vi "Draw_Cage_Outline_(sociability maze).vi"(0 "Picture refnum in":T2, 1 "Bounding rectangle for cage outline, pix (minor)":T1, 2 "Background color":u32(colorbox)=13816530, 3 "Error In":errorcluster) -> (5 "Picture refnum out":T2, 7 "Error Out":errorcluster)   [LabVIEW 2018, in "Cage Diagram.lvlib"]
uses:
  Cage Diagram.lvlib
  <vilib>/vision/Image Controls.llb/IMAQ Image.ctl
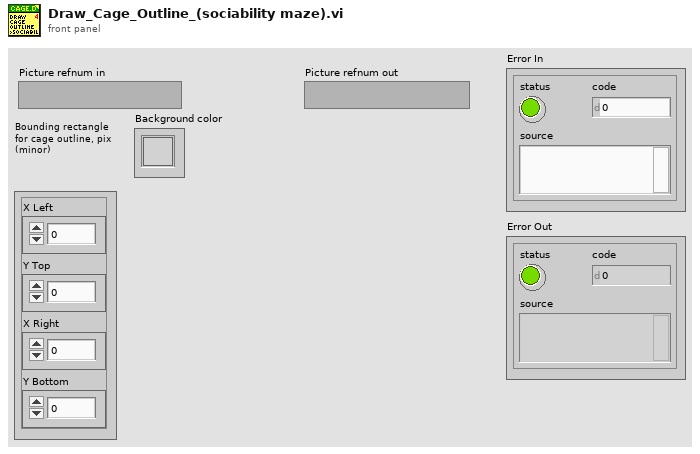
[diagram p1: front panel]
types:
  T1 = cluster{"X Left":i32, "Y Top":i32, "X Right":i32, "Y Bottom":i32}
  T2 = typedef "IMAQ Image.ctl" = refnum<image>
  T3 = cluster{"X Left":dbl, "Y Top":dbl, "X Right":dbl, "Y Bottom":dbl}
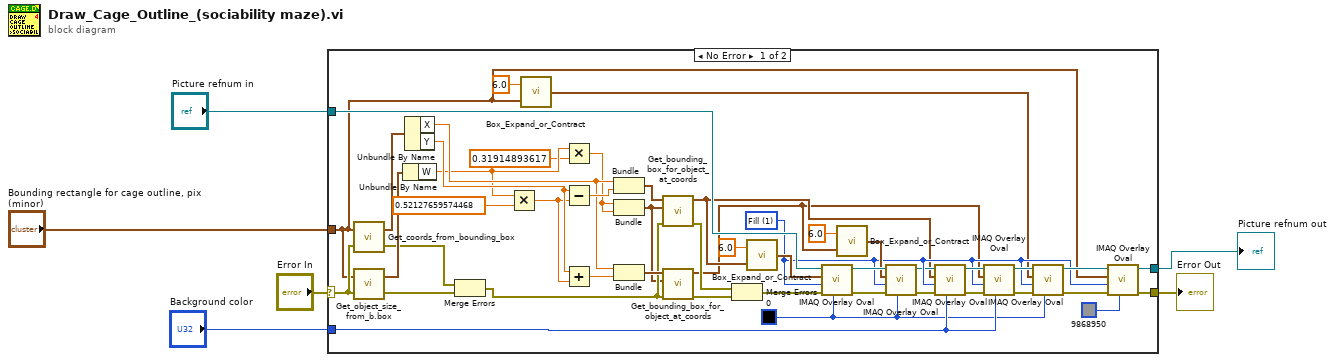
[diagram p0: block diagram]
diagram:
  n1 = case shown="No Error" "Error In" {
    selector: "Error In" -> [w44 w54]
    tunnel: [w28 w55] -> w5
    tunnel: "Picture refnum in" -> [w34 w55]
    tunnel: [w23 w54] -> w3
    tunnel: "Background color" -> [w12 _]
    tunnel: "Bounding rectangle for cage outline, pix (minor)" -> [w7 _]
    frame No Error {
      w9 = u32 0 ("Color")
      w14 = u32 1 items=["Frame", "Fill"] ("Drawing Mode (Frame)")
      n2 = call "Get_coords_from_bounding_box.vi"("Error In"=w44, "Object Bounding Box"=w7) -> ("Error Out"=w43:errorcluster, "Object Coords (center)"=w52:cluster{"X":dbl, "Y":dbl})
      n3 = call "Get_object_size_from_b.box.vi"("Error In"=w44, "Bounding rectangle for cage outline, pix"=w7) -> ("Error Out"=w42:errorcluster, "Object Size, pix"=w53:cluster{"W":dbl, "H":dbl})
      n4 = Unbundle By Name(w53) -> ("W"=w40:dbl)
      n5 = Unbundle By Name(w52) -> ("X"=w45:dbl, "Y"=w50:dbl)
      n6 = Merge Errors(w43, w42) -> (w41:errorcluster)
      n7 = Multiply(x=w40, y=0.52127659574468) -> (x*y=w18:dbl)
      n8 = call "Box_Expand_or_Contract.vi"("Rectangle in"=w7, "Expand/Contract"=6.0) -> ("Rectangle out"=w8:T3)
      n9 = Multiply(x=w40, y=0.31914893617) -> (x*y=w38:dbl)
      n10 = Subtract(x=w50, y=w18) -> (x-y=w49:dbl)
      n11 = Add(x=w50, y=w18) -> (x+y=w46:dbl)
      n12 = Bundle("X"=w45, w49) -> (w48:cluster{"X":dbl, dbl})  [unwired: 1 in]
      n13 = Bundle(w38, w38) -> (w37:cluster{dbl, dbl})  [unwired: 1 in]
      n14 = Bundle("X"=w45, w46) -> (w47:cluster{"X":dbl, dbl})  [unwired: 1 in]
      n15 = call "Get_bounding_box_for_object_at_coords.vi"("Error In"=w41, "Object Size, pix"=w37, "Object Coords, pix"=w48) -> ("Error Out"=w36:errorcluster, "Object Bounding Box"=w11:T3)  [unwired: 7 in]
      n16 = call "Get_bounding_box_for_object_at_coords.vi"("Error In"=w41, "Object Size, pix"=w37, "Object Coords, pix"=w47) -> ("Error Out"=w35:errorcluster, "Object Bounding Box"=w10:T3)  [unwired: 7 in]
      n17 = Merge Errors(w36, w35) -> (w33:errorcluster)
      n18 = call "Box_Expand_or_Contract.vi"("Rectangle in"=w11, "Expand/Contract"=6.0) -> ("Rectangle out"=w17:T3)
      n19 = call "IMAQ Overlay Oval"("Color"=w9, "error in (no error)"=w33, "Drawing Mode (Frame)"=w14, "Bounding Rectangle"=w17, "Image"=w34) -> ("error out"=w27:errorcluster, "Image Out"=w32:T2)  [unwired: 5 in]
      n20 = call "Box_Expand_or_Contract.vi"("Rectangle in"=w10, "Expand/Contract"=6.0) -> ("Rectangle out"=w16:T3)
      n21 = call "IMAQ Overlay Oval"("Color"=w9, "error in (no error)"=w27, "Drawing Mode (Frame)"=w14, "Bounding Rectangle"=w16, "Image"=w32) -> ("error out"=w15:errorcluster, "Image Out"=w13:T2)  [unwired: 5 in]
      n22 = call "IMAQ Overlay Oval"("Color"=w12, "error in (no error)"=w15, "Drawing Mode (Frame)"=w14, "Bounding Rectangle"=w11, "Image"=w13) -> ("error out"=w26:errorcluster, "Image Out"=w31:T2)  [unwired: 5 in]
      n23 = call "IMAQ Overlay Oval"("Color"=w12, "error in (no error)"=w26, "Drawing Mode (Frame)"=w14, "Bounding Rectangle"=w10, "Image"=w31) -> ("error out"=w25:errorcluster, "Image Out"=w29:T2)  [unwired: 5 in]
      n24 = call "IMAQ Overlay Oval"("Color"=w9, "error in (no error)"=w25, "Drawing Mode (Frame)"=w14, "Bounding Rectangle"=w8, "Image"=w29) -> ("error out"=w24:errorcluster, "Image Out"=w30:T2)  [unwired: 5 in]
      n25 = call "IMAQ Overlay Oval"("Color"=u32 9868950, "error in (no error)"=w24, "Drawing Mode (Frame)"=w14, "Bounding Rectangle"=w7, "Image"=w30) -> ("error out"=w23:errorcluster, "Image Out"=w28:T2)  [unwired: 5 in]
    }
    frame Error {
    }
  }
  "Error Out" <- w3
  "Picture refnum out" <- w5
